vi "PH_Synchrolock_Watch.Action Get data.vi"(0 "i ref in":refnum<vi>, 5 "error IO":errorcluster) -> (14 "i ref out":refnum<vi>, 19 "error out":errorcluster)   [LabVIEW 2014, in "PH_Synchrolock_Watch.lvlib"]
doc: "This is the action within the proc case \"Get Data\": The data are analysied and indicated."
uses:
  PH_Synchrolock_Watch.lvlib
  <vilib>/Analysis/baseanly.llb/Mean (DBL).vi
  PH_Devices/PH_TKTDS-30xx/PH_TKTDS-30xx.lvlib
  <vilib>/Analysis/NI_AALBase.lvlib
panel:
  out "something fetched?":bool
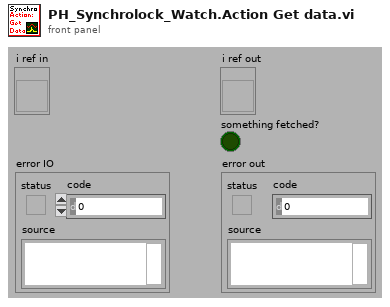
[diagram p1: front panel]
types:
  T1 = typedef "PH_TKTDS-30xx.lvlib/PH_TKTDS-30xx.i attribute.ctl" = cluster{"Default VISA Resource":string, "VISA Resource Name":refnum<visa-resource-name>, "Revision":cluster{"Instrument Driver":string, "Instrument Firmware":string}, "Selftest":cluster{"Result":u32, "Message":string}, "Channels":T2[], "Trigger Configuration":T3, "Acquisition Configuration":T4, "Fetched Waveforms":T5[], "GUI Refs":T6, "GUI Refs Channels":refnum<vi>[], "State":T7, "Error Message":string, "Allow Prdc Loop?":bool}
  T2 = typedef "PH_TKTDS-30xx.lvlib/PH_TKTDS-30xx.Channel Config.ctl" = cluster{"Channel Name":string, "Input Impedance":string, "Max Input Frequency":string, "Vertical Coupling":i32, "Channel Enabled":bool, "Probe Attenuation":dbl, "Vertical Range":dbl, "Vertical Offset":dbl}
  T3 = typedef "PH_TKTDS-30xx.lvlib/PH_TKTDS-30xx.Trigger Config.ctl" = cluster{"Source":string, "Slope":i32, "Level [V]":dbl}
  T4 = typedef "PH_TKTDS-30xx.lvlib/PH_TKTDS-30xx.Acquisition Config.ctl" = cluster{"Time base":dbl, "Record Length":u16, "Start Time":dbl, "Type":i32, "Continuous":bool}
  T5 = typedef "PH_TKTDS-30xx.lvlib/PH_TKTDS-30xx.fetched Waveform.ctl" = cluster{"Source":string, "Actual Points":u32, "Initial X":dbl, "X Increment":dbl, "Waveform Array":dbl[]}
  T6 = typedef "PH_TKTDS-30xx.lvlib/PH_TKTDS-30xx.GUI Refs.ctl" = cluster{"Trigger":refnum<vi>, "Acquisition":refnum<vi>, "Graph":refnum<vi>, "State":refnum<vi>, "Delete":refnum<vi>, "Channel to be positioned":refnum<vi>, "Postion":refnum<vi>, "Display Intensity":refnum<vi>, "VISA Resource":refnum<vi>}
  T7 = typedef "PH_StatusHandler.lvlib/PH_StatusHandler.Status.ctl" = i16
  T8 = typedef "PH_Synchrolock_Watch.lvlib/PH_Synchrolock_Watch.i attribute.ctl" = cluster{"GUI Refs":cluster{"Mean Phase Graph":refnum<vi>, "RF Amplitude Graph":refnum<vi>, "Mira Amplitude Graph":refnum<vi>, "MIRA State":refnum<vi>, "Mean Phase":refnum<vi>, "RF Amplitude":refnum<vi>, "Mira Amplitude":refnum<vi>, "Mean Phase in range?":refnum<vi>, "RF Amplitude above limit?":refnum<vi>, "Mira Amplitude in range?":refnum<vi>, "Mean phase upper limit":refnum<vi>, "Mean phase lower limit":refnum<vi>, "RF Amplitude lower limit":refnum<vi>, "Mira Amplitude lower limit":refnum<vi>, "Mira Amplitude upper limit":refnum<vi>, "Waveform End":refnum<vi>, "Mira scope":refnum<vi>, "Reset Mira warning":refnum<vi>}, "Status":cluster{"Reset Warning":bool}, "Mean Phase":cluster{"Current Value":dbl, "Upper Limit":dbl, "Lower Limit":dbl, "Data":cluster{dbl[], dbl[]}}, "RF":cluster{"Current Value":dbl, "Lower Limit":dbl, "Data":cluster{dbl[], dbl[]}}, "MIRA":cluster{"Current Value":dbl, "Upper Limit":dbl, "Lower Limit":dbl, "Data":cluster{dbl[], dbl[]}}, "Waveform End":i32}
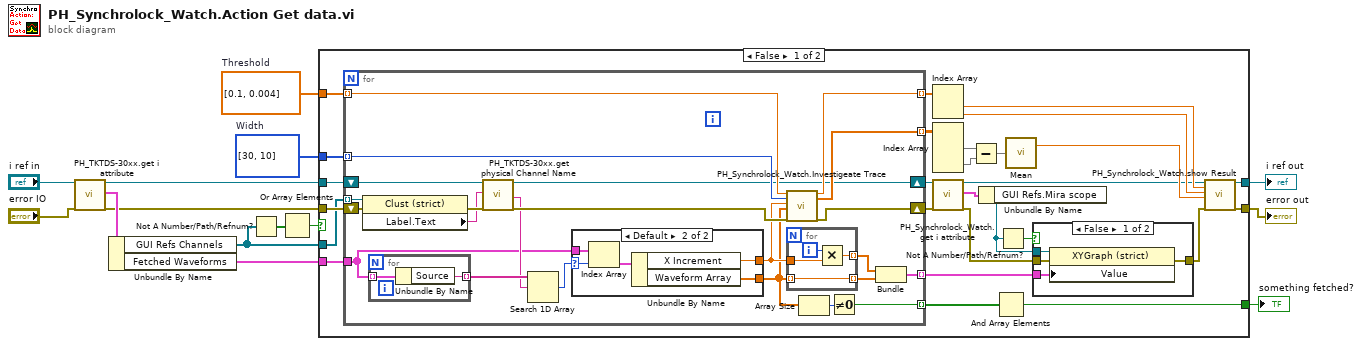
[diagram p0: block diagram]
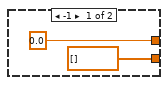
[diagram p2: hidden frame]
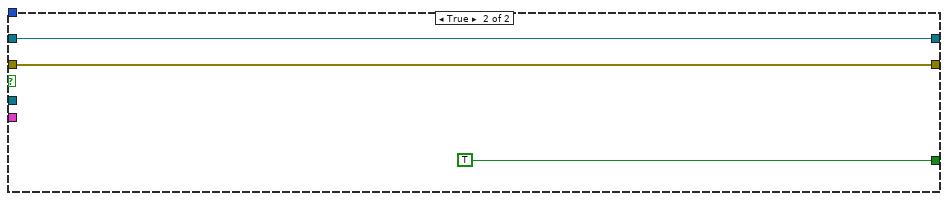
[diagram p4: hidden frame]
diagram:
  w5 = dbl[] [0.1, 0.004]  # Threshold
  w4 = i32[] [30, 10]  # Width
  n1 = call "PH_TKTDS-30xx.get i attribute.vi"("i ref in"="i ref in", "error in (no error)"="error IO") -> ("i ref out"=w12:refnum<vi>, "i attribute"=w13:T1, "error out"=w11:errorcluster)  [unwired: 15 in]
  n2 = Unbundle By Name(w13) -> ("GUI Refs Channels"=w6:refnum<vi>[], "Fetched Waveforms"=w14:T5[])
  n3 = Not A Number/Path/Refnum?(number/path/refnum=w6) -> (NaN/Path/Refnum?=w8:bool[])
  n4 = Or Array Elements(Boolean array=w8) -> (logical OR=w7:bool)
  n5 = case shown="False" w7 {
    tunnel: w14 -> [w41 _]
    tunnel: w12 -> [w28 w85]
    tunnel: w11 -> [w39 w84]
    tunnel: [w34 w85] -> w10
    tunnel: [w33 w84] -> w9
    tunnel: w6 -> [w29 _]
    tunnel: w5 -> [w27 _]
    tunnel: w4 -> [w26 _]
    tunnel: [w15 TRUE] -> w1
    frame False {
      n6 = for {
        tunnel: w41 -> [w46]
        tunnel: [w60] -> w18 mode=indexing
        tunnel: w27 -> [w59] mode=indexing
        tunnel: w26 -> [w58] mode=indexing
        shift-right: [w56] -> w21
        shift-left: w39 -> [w57]
        tunnel: [w55] -> w35 mode=indexing
        tunnel: [w54] -> w36 mode=indexing
        tunnel: w29 -> [w53] mode=indexing
        shift-right: [w48] -> w23
        shift-left: w28 -> [w49]
        tunnel: [w42] -> w16 mode=indexing
        n7 = property class="Clust (strict)"(reference=w53, error in=w57) -> (error out=w51:errorcluster, "Label.Text"=w50:string)  [unwired: 1 out]
        n8 = for {
          tunnel: w46 -> [w77] mode=indexing
          tunnel: [w76] -> w63 mode=indexing
          n9 = Unbundle By Name(w77) -> ("Source"=w76:string)
        }
        n10 = call "PH_TKTDS-30xx.get physical Channel Name.vi"("i ref in"=w49, "GUI Element Name"=w50, "error in"=w51) -> ("i ref out"=w48:refnum<vi>, "Physical Channel Name"=w47:string, "error out"=w52:errorcluster)  [unwired: 14 in]
        n11 = Search 1D Array(1D array=w63, element=w47) -> (index of element=w64:i32)  [unwired: 1 in]
        n12 = case shown="Default" w64 {
          selector: w64 -> [_ w71]
          tunnel: w46 -> [_ w75]
          tunnel: [0.0 ("X Increment") w73] -> w45
          tunnel: [dbl[] [] ("Waveform Array") w72] -> w44
          frame -1 {
          }
          frame Default {
            n13 = Index Array(array=w75, index=w71) -> (element=w74:T5)
            n14 = Unbundle By Name(w74) -> ("X Increment"=w73:dbl, "Waveform Array"=w72:dbl[])
          }
        }
        n15 = call "PH_Synchrolock_Watch.Investigeate Trace.vi"("Threshold"=w59, "Width"=w58, "X Increment"=w45, "Waveform Array"=w44, "error in"=w52) -> ("Mean Amplitude"=w55:dbl, "Peak Locations"=w54:dbl[], "error out"=w56:errorcluster)  [unwired: 12 in]
        n16 = for {
          tunnel: w44 -> [w66] mode=indexing
          tunnel: w45 -> [w67]
          tunnel: [w65] -> w62 mode=indexing
          tunnel: [w66] -> w61 mode=indexing
          i -> [w68]
          n17 = Multiply(x=w68, y=w67) -> (x*y=w65:dbl)
        }
        n18 = Array Size(array=w44) -> (size(s)=w43:i32)
        n19 = Not Equal To 0?(x=w43) -> (x != 0?=w42:bool)
        n20 = Bundle(w62, w61) -> (w60:cluster{dbl[], dbl[]})  [unwired: 1 in]
      }
      n21 = Index Array(array=w35) -> (element #1=w31:dbl, element #2=w30:dbl)  [unwired: 2 in]
      n22 = Index Array(array=w36) -> (element #1=w38:dbl[], element #2=w37:dbl[])  [unwired: 4 in]
      n23 = call "PH_Synchrolock_Watch.get i attribute.vi"("i ref in"=w23, "error in (no error)"=w21) -> ("i ref out"=w22:refnum<vi>, "i attribute"=w19:T8, "error out"=w20:errorcluster)  [unwired: 15 in]
      n24 = Subtract(x=w38, y=w37) -> (x-y=w25:dbl[])
      n25 = Unbundle By Name(w19) -> ("GUI Refs.Mira scope"=w17:refnum<vi>)
      n26 = And Array Elements(Boolean array=w16) -> (logical AND=w15:bool)
      n27 = Not A Number/Path/Refnum?(number/path/refnum=w17) -> (NaN/Path/Refnum?=w40:bool)
      n28 = call-poly <vilib>:"Mean.vi"("X"=w25) -> ("mean"=w24:dbl)  [unwired: 1 out]
      n29 = case shown="False" w40 {
        tunnel: w20 -> [w81 w82]
        tunnel: [w80 w82] -> w32
        tunnel: w17 -> [w79 _]
        tunnel: w18 -> [w78 _]
        frame False {
          n30 = property class="XYGraph (strict)"(reference=w79, error in=w81, "Value"=w78) -> (error out=w80:errorcluster)  [unwired: 1 out]
        }
        frame True {
        }
      }
      n31 = call "PH_Synchrolock_Watch.show Result.vi"("i ref in"=w22, "RF Current Value"=w31, "Mira Current Value"=w30, "Mean Phase Current Value"=w24, "error in"=w32) -> ("i ref out"=w34:refnum<vi>, "error out"=w33:errorcluster)  [unwired: 13 in]
    }
    frame True {
    }
  }
  "error out" <- w9
  "i ref out" <- w10
  "something fetched?" <- w1
